vi "wrap.CurrentLine.vi"(0 "class.GLue in":refnum<class "class.GLue.lvclass">, 7 "Value in":i32, 11 "error in (no error)":errorcluster, 13 "Write?":bool) -> (4 "class.GLue out":refnum<class "class.GLue.lvclass">, 8 "Value out":i32, 15 "error out":errorcluster)   [LabVIEW 2014, in "GLue.lvlib" / "class.GLue.lvclass"]
uses:
  class.GLue.lvclass
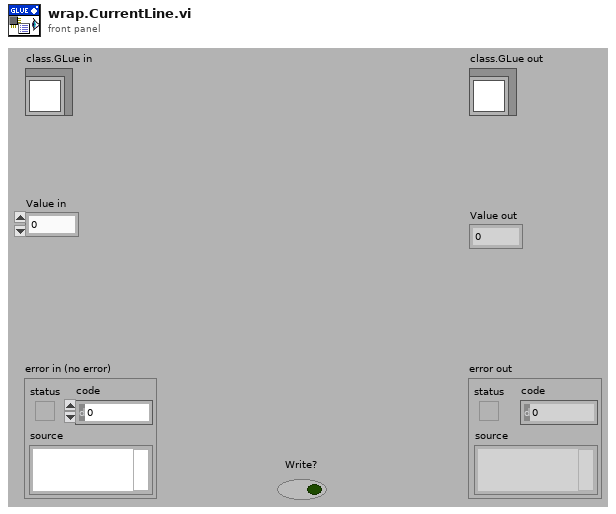
[diagram p1: front panel]
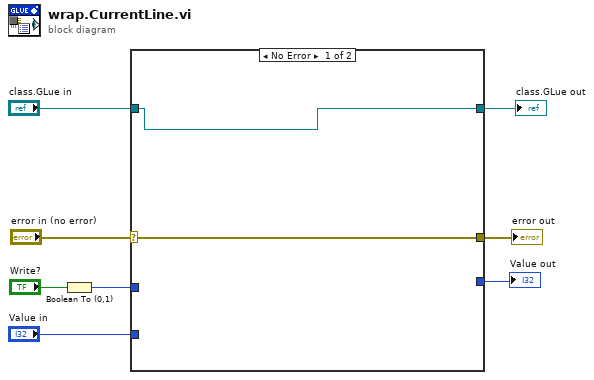
[diagram p0: block diagram]
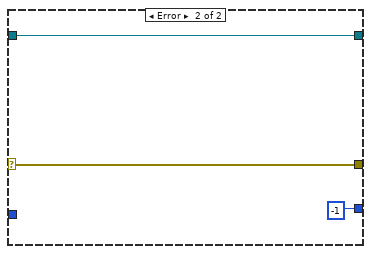
[diagram p2: hidden frame]
diagram:
  n1 = Boolean To (0,1)(Boolean="Write?") -> (0, 1=w1:i16)
  n2 = case shown="No Error" "error in (no error)" {
    selector: "error in (no error)" -> [w9 w13]
    tunnel: [w9 w13] -> w7
    tunnel: [w10 w12] -> w5
    tunnel: "class.GLue in" -> [w10 w12]
    tunnel: [_ -1 ("TopType")] -> w4
    tunnel: "Value in" -> [_ _]
    tunnel: w1 -> [_ _]
    frame No Error {
    }
    frame Error {
    }
  }
  "error out" <- w7
  "class.GLue out" <- w5
  "Value out" <- w4
